vi "VolumeDescriptor+File reference.vi"(8 "error in (no error)":errorcluster, 11 "VGS_VolumeDescriptor+File in":refnum<class "VGS_VolumeDescriptor+File.lvclass">) -> (0 "error out":errorcluster, 2 "VolumeDescriptor+File":refnum<k24>, 3 "VGS_VolumeDescriptor+File out":refnum<class "VGS_VolumeDescriptor+File.lvclass">)   [LabVIEW 2022 SP3, in "LV_VGS.lvlib" / "VGS_VolumeDescriptor+File.lvclass"]
uses:
  VGS_VolumeDescriptor+File.lvclass
  C:/Users/Andrey/Documents/GitHub/LV_VGS/vgs_project.dll
  vgs_project.dll
  VGS_VolumeDescriptor+File.lvclass/VGS_VolumeDescriptor+File.ctl
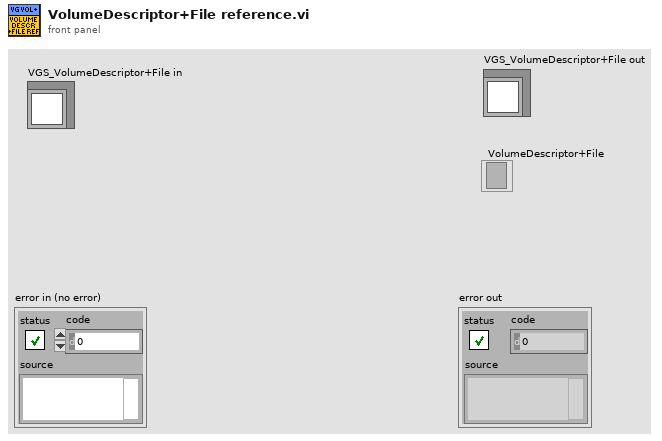
[diagram p1: front panel]
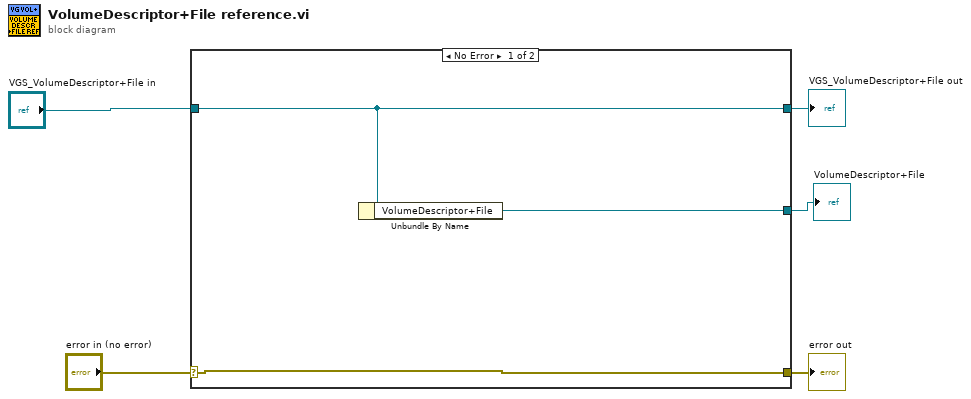
[diagram p0: block diagram]
diagram:
  n1 = case shown="No Error" "error in (no error)" {
    selector: "error in (no error)" -> [w7 w10]
    tunnel: [w7 w10] -> w4
    tunnel: [w6 w9] -> w2
    tunnel: "VGS_VolumeDescriptor+File in" -> [w6 w9]
    tunnel: [w8 _] -> w1
    frame No Error {
      n2 = Unbundle By Name(w6) -> ("VolumeDescriptor+File"=w8:refnum<k24>)
    }
    frame Error {
    }
  }
  "error out" <- w4
  "VGS_VolumeDescriptor+File out" <- w2
  "VolumeDescriptor+File" <- w1
